vi "onAssertionSlippage.vi"(7 "AssertCompareValue in":refnum<class "AssertCompareValue.lvclass">, 11 "Leaf.Assertion":refnum<class "Leaf.Assertion.lvclass">) -> (0 "error out":errorcluster, 3 "Leaf.Assertion":refnum<class "Leaf.Assertion.lvclass">)   [LabVIEW 2021, in "Bananas.lvlib" / "AssertCompareValue.lvclass"]
uses:
  AssertCompareValue.lvclass
  Leaf.Assertion/Leaf.Assertion.lvclass
  C:/Repositories/LVOS/Bananas/lv-src/Bananas/Leaf/Leaf.lvclass
  AssertCompareValue.lvclass/AssertCompareValue.ctl
  Read Greater_.vi
  Read Equal_.vi
  Read X.vi
  Read Y.vi
  <vilib>/LabVIEW Open Source Project/Data Manipulation/Variant/OpenVariant.lvlib
  Leaf/Leaf.lvclass
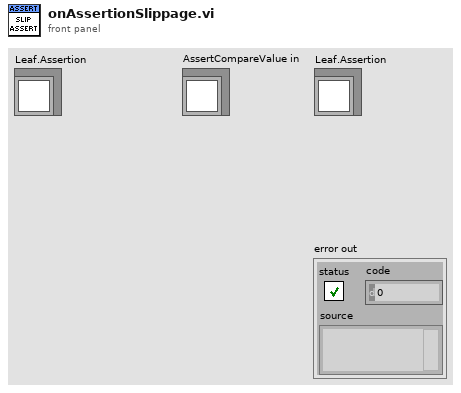
[diagram p1: front panel]
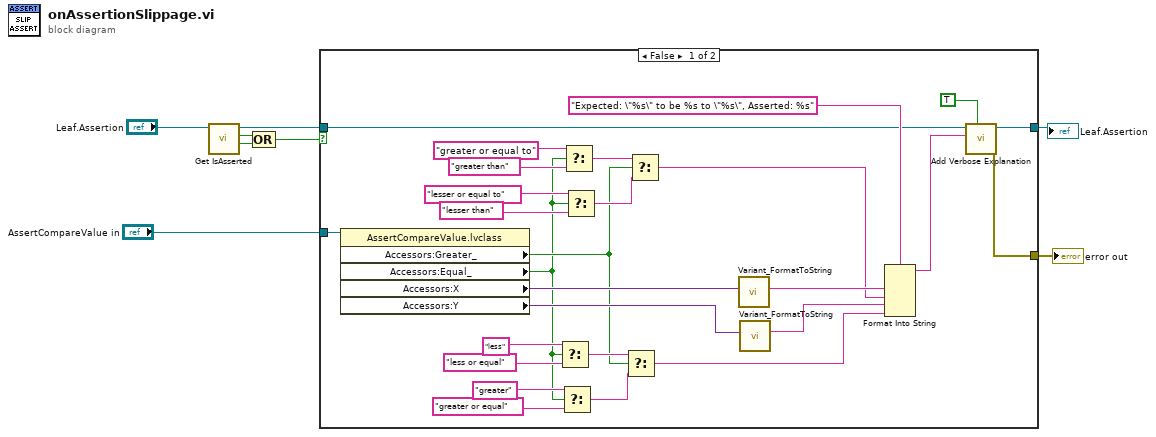
[diagram p0: block diagram]
diagram:
  n1 = call "Get IsAsserted.vi"("Leaf.Assertion"="Leaf.Assertion") -> ("Skipped"=w2:bool, "Asserted"=w3:bool, "Leaf.Assertion"=w1:refnum<class "Leaf.Assertion.lvclass">)  [unwired: 8 in]
  n2 = Compound Arithmetic op=OR(w3, w2) -> (w8:bool)
  n3 = case shown="False" w8 {
    tunnel: [w12 w36] -> w7
    tunnel: [w9 _] -> w6
    tunnel: w1 -> [w13 w36]
    tunnel: "AssertCompareValue in" -> [w35 _]
    frame False {
      n4 = property class="AssertCompareValue.lvclass"(reference=w35) -> ("Accessors:Greater_"=w17:bool, "Accessors:Equal_"=w16:bool, "Accessors:X"=w34:variant, "Accessors:Y"=w33:variant)  [unwired: 1 in, 2 out]
      n5 = Select(t="less", s=w16, f="less or equal" ("t")) -> (s? t:f=w20:string)
      n6 = Select(t="greater", s=w16, f="greater or equal" ("t")) -> (s? t:f=w22:string)
      n7 = Select(t="greater or equal to", s=w16, f="greater than" ("t")) -> (s? t:f=w28:string)
      n8 = Select(t="lesser or equal to", s=w16, f="lesser than" ("t")) -> (s? t:f=w25:string)
      n9 = Select(t=w20, s=w17, f=w22) -> (s? t:f=w15:string)
      n10 = Select(t=w28, s=w17, f=w25) -> (s? t:f=w31:string)
      n11 = call <vilib>:"Variant_FormatToString.vi"("Variant"=w34) -> ("Value"=w32:string)  [unwired: 10 in]
      n12 = call <vilib>:"Variant_FormatToString.vi"("Variant"=w33) -> ("Value"=w24:string)  [unwired: 10 in]
      n13 = Format Into String(format string="Expected: \"%s\" to be %s to \"%s\", Asserted: %s" ("t"), w32, w31, w24, w15) -> (resulting string=w10:string)  [unwired: 2 in, 1 out]
      n14 = call "Add Verbose Explanation.vi"("overwrite"=TRUE ("overwrite?"), "Verbose Explanation"=w10, "Leaf in"=w13) -> ("error out"=w9:errorcluster, "Leaf out"=w12:refnum<class "Leaf.Assertion.lvclass">)  [unwired: 7 in]
    }
    frame True {
      # "There was an upstream error or the assertion = TRUE"
    }
  }
  "error out" <- w6
  "Leaf.Assertion" <- w7
